vi "Explain error.vi"(1 "error":u32) -> (0 "error string":string)   [LabVIEW 2013]
uses:
  lib/FTCSPI.dll
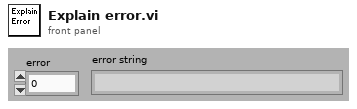
[diagram p1: front panel]
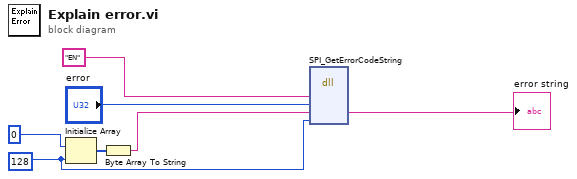
[diagram p0: block diagram]
diagram:
  w1 = 128
  n1 = Initialize Array(u8 0 ("element"), w1) -> (w3:u8[])
  n2 = Byte Array To String(unsigned byte array=w3) -> (string=w2:string)
  n3 = dll-call lib="C:/Users/SuperUser/Documents/HiSparc/hisparcdaq/FPGA/lib/FTCSPI.dll" fn="SPI_GetErrorCodeString"("language"="EN", "status"="error", "buffer"=w2, "size"=w1) -> ("buffer"=→"error string":string)  [unwired: 4 in, 5 out]
